vi "Wheel of Doom Internal Global.vi"() -> ()   [LabVIEW 2019]
panel:
  out "Shooting":bool
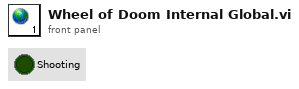
[diagram p1: front panel]
diagram:
